vi "FPGA Personality.vi"   [LabVIEW 2015]
doc: "This VI generates a sine waveform with an FPGA target. The waveform numeric data is output via DMA Target to Host FIFO."
uses:
  <vilib>/rvi/Emulation/niFpgaGetClockAttributes.vi
  <vilib>/rvi/Emulation/niFpgaSctlEmulationGetInTimedLoop.vi
  <vilib>/rvi/Emulation/niFpgaEmulationReportErrorSimple.vi
  <vilib>/rvi/interface/RandomDataEmulation/niFpgaRandomDataHandleErrors.vi
  <vilib>/rvi/Emulation/niFpgaCriticalErrorInLSC.vi
  <vilib>/rvi/DataTransferAndStorage/Container/XNode/niFpgaContainer.xnode
  <vilib>/rvi/interface/RandomDataEmulation/nirviRandomDataFpgaReadWriteTemplate.vi
panel:
  # "This VI generates a sine waveform of a fixed frequency on the FPGA. \nThe waveform numeric data is output via Direct Memory Access (DMA) \nTarget to Host FIFO, which you will read in the real-time TCP File Sender VI."
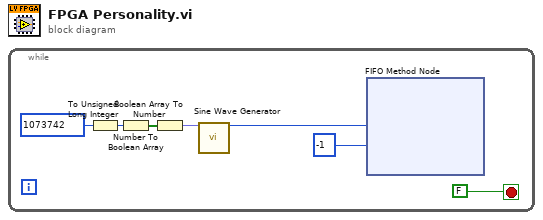
[diagram p0: block diagram]
diagram:
  n1 = while {
    stop <- FALSE ("stop") stop-if-true
    n2 = To Unsigned Long Integer(number=u32 1073742 ("phase increment")) -> (unsigned 32bit integer=w5:u32)
    n3 = Number To Boolean Array(number=w5) -> (Boolean array=w3:bool[])
    n4 = Boolean Array To Number(Boolean array=w3) -> (number=w4:fxp<+,32,0>)
    n5 = call "Sine Wave Generator"("frequency (periods/tick)"=w4) -> ("sine out"=w1:i16)  [unwired: 14 in]
    n6 = xnode "FIFO Method Node"("Element"=w1, "Timeout"=-1) -> ()  [unwired: 1 in, 2 out]
  }
